vi "SPC_read_data_frame.vi"(6 "Input Buffer":u16[](array[numeric]), 7 "Frame":i32 min=0 max=65535 step=1, 8 "Error In":errorcluster, 9 "Page":i32 min=0 max=65535 step=1, 10 "Module No":i16 min=0 max=7 step=1, 11 "DLL Path":path) -> (0 "Error Out":errorcluster, 2 "Module No":i16 min=0 max=7 step=1, 3 "DLL Path":path, 4 "Output Data":u16[](array[numeric]))   [LabVIEW 2023]
doc: "The procedure reads data from a frame of the SPC memory on module 'mod_no' defined by the parameters 'frame' and 'page' to the buffer 'data'. The procedure is used to read measurement results from the SPC memory when frames_per_page is greater than 1 (this can be the case for SPC7x0/830/140 modules in scanning modes).\nThe range of the parameters 'frame' and 'page' depends on the actual configuration of the SPC memory (see SPC_configure_memory).\nIf 'frame' is equal -1, all frames(frames_per_page) from the page 'page' are read.\nTo provide correct access to the SPC memory it is required that the function SPC_configure_memory be used( in normal operation modes) before the first call of SPC_read_data_frame. This function also delivers the required information about the block/page structure of the SPC memory:\nlong max_block_no total number of blocks (=curves) in the memory ( memory bank for the SPC- 6x0/13x/15x/160)\nlong blocks_per_frame Number of blocks (=curves) per frame\nlong frames_per_page Number of frames per page\nlong maxpage max number of pages to use in a measurement\nlong block_length Number of 16-bits words per one block (curve)\nPlease make sure that the buffer 'data' be allocated with enough memory for \nblock_length * blocks_per_frame 16-bit values, when one frame is read, or \nblock_length * blocks_per_frame * frames_per_page 16-bit values, when 'frame' = -1.\n\ninfo@becker-hickl.com"
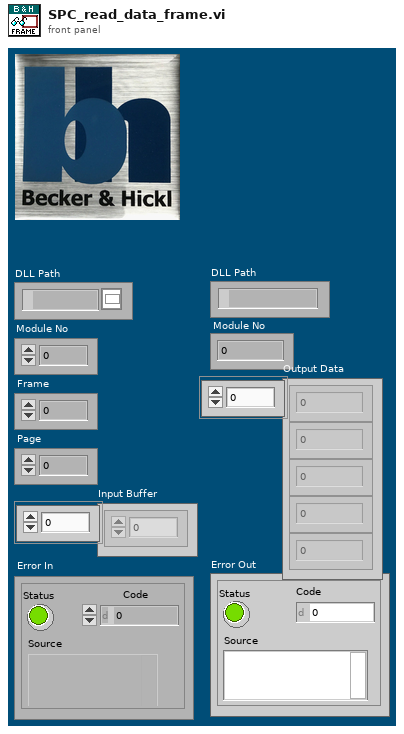
[diagram p1: front panel]
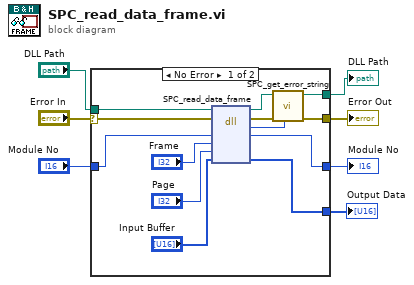
[diagram p0: block diagram]
diagram:
  n1 = case shown="No Error" "Error In" {
    selector: "Error In" -> [w15 w23]
    tunnel: [w17 w23] -> w7
    tunnel: [w13 w22] -> w6
    tunnel: "DLL Path" -> [w16 w22]
    tunnel: "Module No" -> [w11 w21]
    tunnel: [w10 w21] -> w2
    tunnel: [w8 _] -> w1
    frame No Error {
      n2 = dll-call lib="D:/spcm/lib/lab_view/lv10.0/spcm32.dll" fn="SPC_read_data_frame"(path in=w16, error in=w15, "mod_no"=w11, "frame"="Frame", "page"="Page", "data"="Input Buffer") -> (path out=w14:path, error out=w18:errorcluster, "return type"=w12:i16, "mod_no"=w10:i16, "data"=w8:u16[])  [unwired: 3 in]
      n3 = call "SPC_get_error_string.vi"("ErrorID"=w12, "Error In"=w18, "DLL Path"=w14) -> ("Error Out"=w17:errorcluster, "DLL Path"=w13:path)  [unwired: 6 in, 1 out]
    }
    frame Error {
    }
  }
  "DLL Path" <- w6
  "Error Out" <- w7
  "Module No" <- w2
  "Output Data" <- w1
